vi "rad7_subviv2.vi"(8 "error in (no error)":errorcluster, 10 "Slow control read rate (Hz)":dbl=1.0, 11 "VISA resource name":refnum<visa-resource-name>) -> (0 "error out":errorcluster, 1 "Buffer length":u32, 2 "Rad7 data out":string, 3 "VISA resource name out":refnum<visa-resource-name>, 4 "Erase done?":bool)   [LabVIEW 2012]
uses:
  <vilib>/Instr/_visa.llb/VISA Configure Serial Port (Instr).vi
panel:
  out "Enum":T1(ring)
  out "Numeric 2":i32
  out "read buffer":string
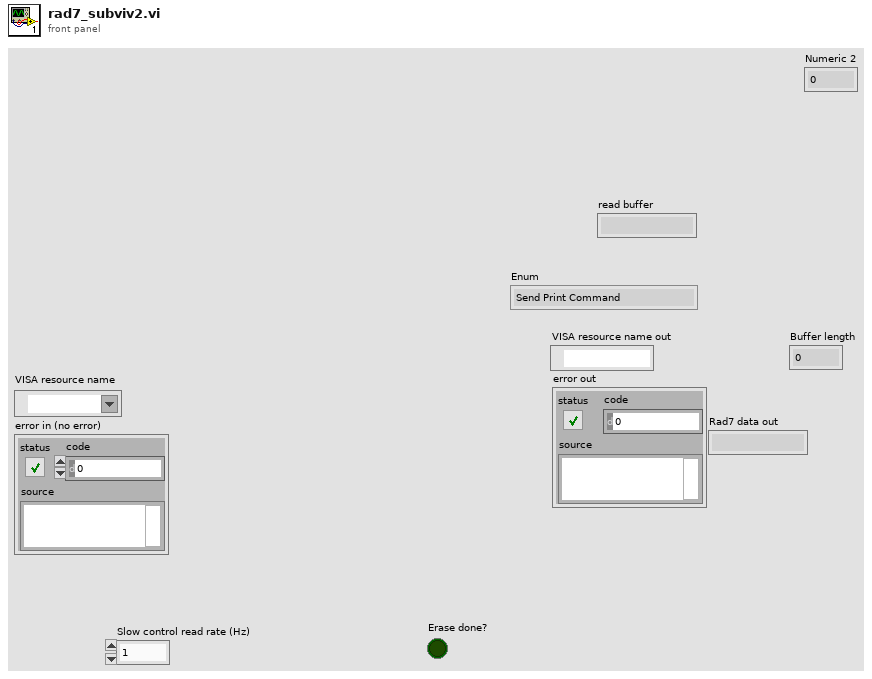
[diagram p1: front panel]
types:
  T1 = enum16{"Send Print Command", "Wait 5 seconds", "Remove first junk characters", "Data good?", "Read Buffer", "Wait 1 second", "Erase data from Rad7", "Confirm", "Error"}
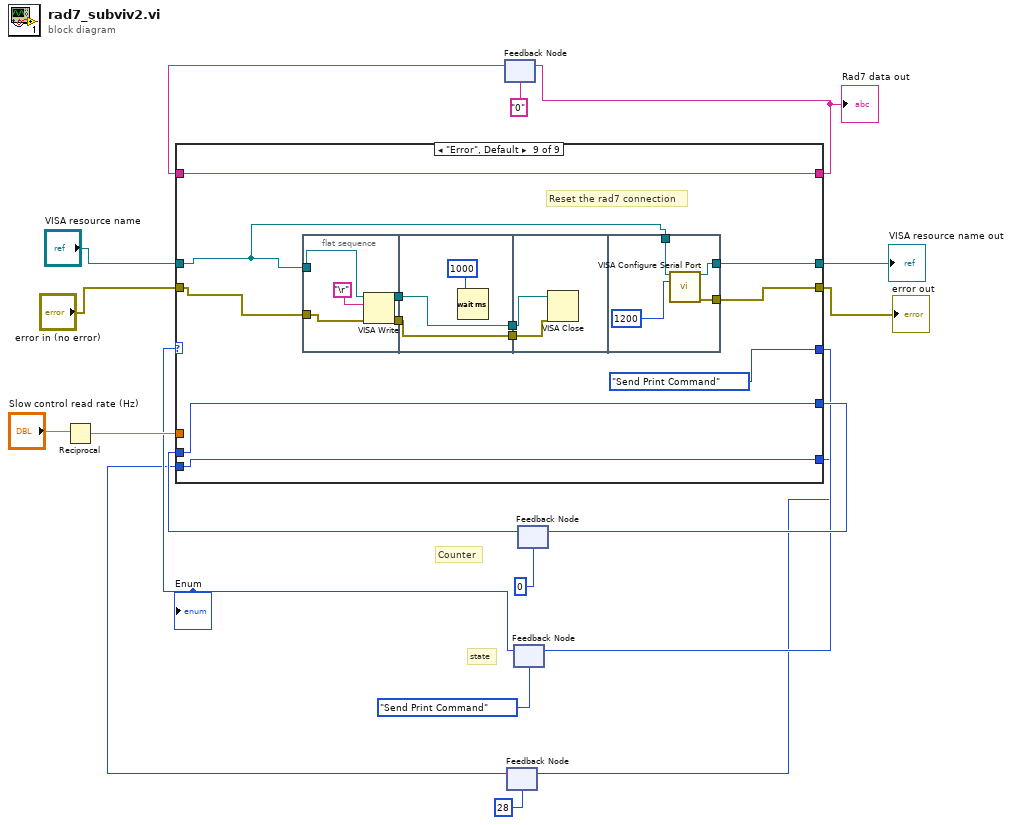
[diagram p0: block diagram]
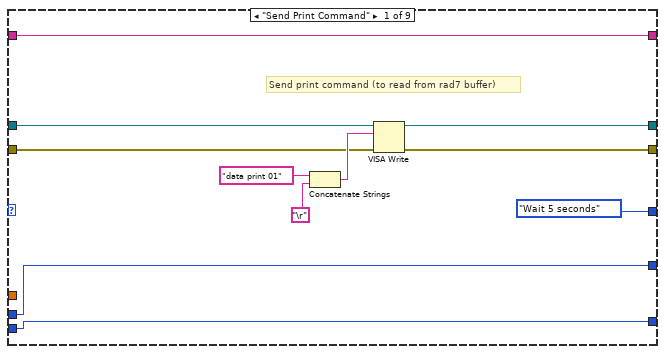
[diagram p2: hidden frame]
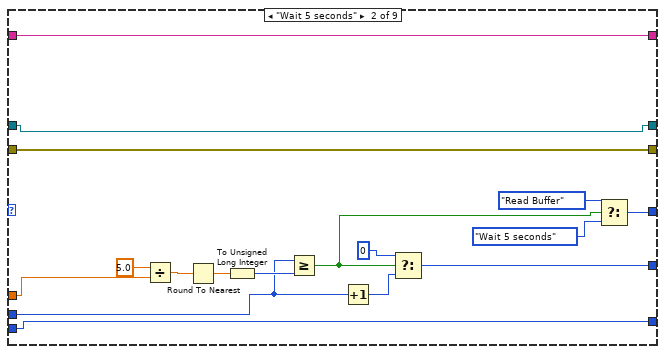
[diagram p3: hidden frame]
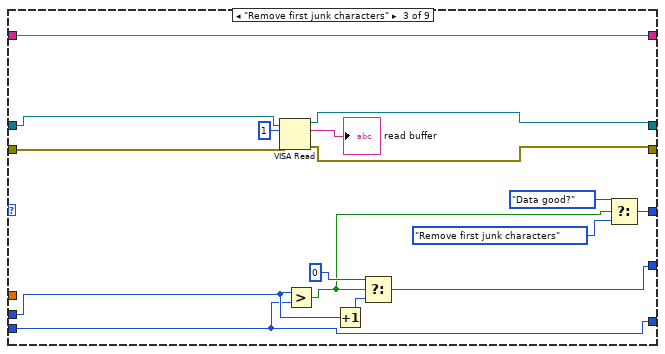
[diagram p4: hidden frame]
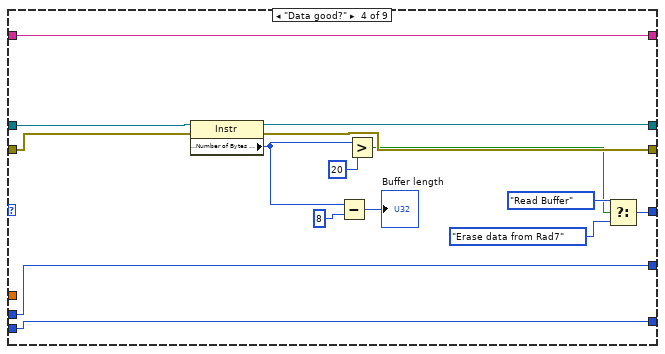
[diagram p5: hidden frame]
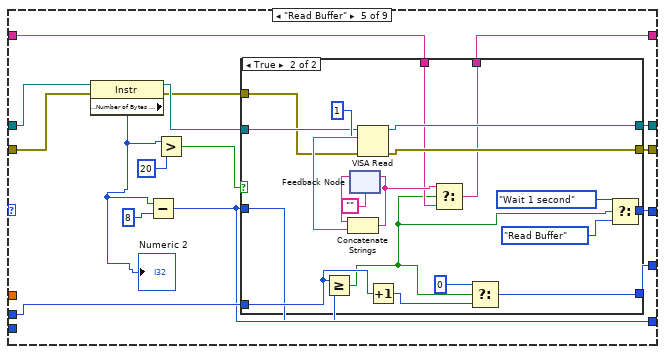
[diagram p6: hidden frame]
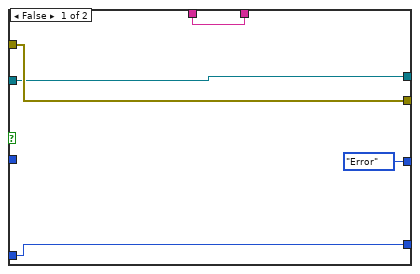
[diagram p7: hidden frame]
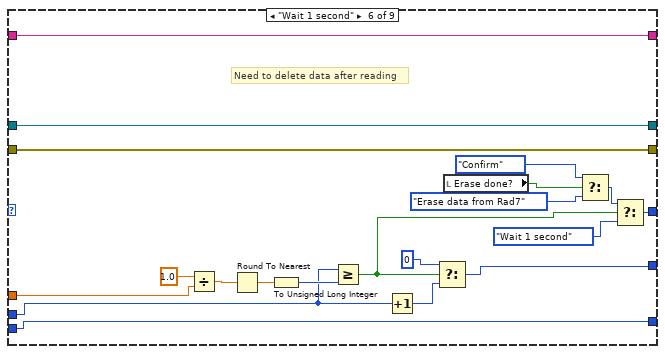
[diagram p8: hidden frame]
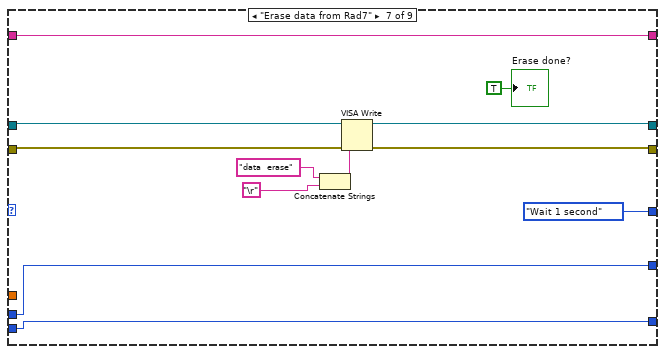
[diagram p9: hidden frame]
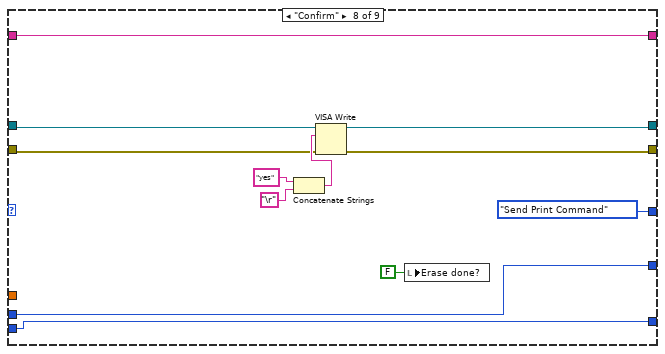
[diagram p10: hidden frame]
diagram:
  # "state"
  # "Counter"
  n1 = Reciprocal(x="Slow control read rate (Hz)") -> (1/x=w12:dbl)
  n2 = feedback #1("0") -> (w9:string)
  n3 = feedback #2(u32 28 ("y")) -> (w2:u32)
  n4 = feedback #3(T1."Send Print Command" ("Enum")) -> (w6:T1)
  "Enum" <- w6
  n5 = feedback #4(u32 0) -> (w11:u32)
  n6 = case shown="\"Error\", Default" w6 {
    tunnel: [T1."Wait 5 seconds" ("Enum") w44 w60 w75 w93 w136 T1."Wait 1 second" ("Enum") T1."Send Print Command" ("Enum") T1."Send Print Command" ("Enum")] -> w5
    tunnel: "VISA resource name" -> [w25 w32 w53 w69 w84 w125 w145 w157 w165]
    tunnel: [w24 w32 w51 w67 w92 w125 w143 w155 w164] -> w14
    tunnel: "error in (no error)" -> [w23 w31 w52 w68 w82 w124 w144 w156 w166]
    tunnel: [w22 w31 w50 w66 w91 w124 w142 w154 w163] -> w13
    tunnel: w12 -> [_ w39 _ _ _ w127 _ _ _]
    tunnel: w11 -> [w21 w37 w57 w74 w90 w130 w140 w153 w173]
    tunnel: [w21 w36 w56 w74 w89 w129 w140 w153 w173] -> w10
    tunnel: w9 -> [w20 w33 w49 w64 w87 w126 w141 w152 w172]
    tunnel: [w20 w33 w49 w64 w88 w126 w141 w152 w172] -> w8
    tunnel: w2 -> [w19 w30 w47 w63 _ w119 w139 w151 w171]
    tunnel: [w19 w30 w47 w63 w79 w119 w139 w151 w171] -> w1
    frame "Send Print Command" {
      # "Send print command (to read from rad7 buffer)"
      n7 = Concatenate Strings("data print 01" ("Command"), "\r") -> (w28:string)
      n8 = VISA Write(VISA resource name=w25, write buffer=w28, error in (no error)=w23) -> (VISA resource name out=w24:refnum<visa-resource-name>, error out=w22:errorcluster)  [unwired: 1 out]
    }
    frame "Wait 5 seconds" {
      n9 = Divide(x=5.0, y=w39) -> (x/y=w43:dbl)
      n10 = Round To Nearest(number=w43) -> (nearest integer value=w42:dbl)
      n11 = To Unsigned Long Integer(number=w42) -> (unsigned 32bit integer=w41:u32)
      n12 = Greater Or Equal?(x=w37, y=w41) -> (x >= y?=w34:bool)
      n13 = Increment(x=w37) -> (x+1=w40:u32)
      n14 = Select(t=u32 0, s=w34, f=w40) -> (s? t:f=w36:u32)
      n15 = Select(t=T1."Read Buffer" ("Enum"), s=w34, f=T1."Wait 5 seconds" ("Enum")) -> (s? t:f=w44:T1)
    }
    frame "Remove first junk characters" {
      n16 = VISA Read(VISA resource name=w53, byte count=u32 1, error in (no error)=w52) -> (VISA resource name out=w51:refnum<visa-resource-name>, read buffer=→"read buffer":string, error out=w50:errorcluster)  [unwired: 1 out]
      n17 = Greater?(x=w57, y=w47) -> (0:w48:bool)
      n18 = Increment(x=w57) -> (x+1=w59:u32)
      n19 = Select(t=u32 0, s=w48, f=w59) -> (s? t:f=w56:u32)
      n20 = Select(t=T1."Data good?" ("Enum"), s=w48, f=T1."Remove first junk characters" ("Enum")) -> (s? t:f=w60:T1)
    }
    frame "Data good?" {
      n21 = property class="Instr"(reference=w69, error in=w68) -> (reference out=w67:refnum<visa-resource-name>, error out=w66:errorcluster, "Serial Settings:Number of Bytes at Serial Port"=w71:u32)
      n22 = Subtract(x=w71, y=u32 8) -> (x-y=→"Buffer length":u32)
      n23 = Greater?(x=w71, y=u32 20) -> (0:w65:bool)
      n24 = Select(t=T1."Read Buffer" ("Enum"), s=w65, f=T1."Erase data from Rad7" ("Enum")) -> (s? t:f=w75:T1)
    }
    frame "Read Buffer" {
      n25 = property class="Instr"(reference=w84, error in=w82) -> (reference out=w83:refnum<visa-resource-name>, error out=w81:errorcluster, "Serial Settings:Number of Bytes at Serial Port"=w80:u32)
      "Numeric 2" <- w80
      n26 = Subtract(x=w80, y=8) -> (x-y=w79:u32)
      n27 = Greater?(x=w80, y=20) -> (0:w78:bool)
      n28 = case shown="True" w78 {
        tunnel: [T1."Error" ("Enum") w116] -> w93
        tunnel: [w96 w111] -> w92
        tunnel: [w97 w110] -> w91
        tunnel: w90 -> [w95 w107]
        tunnel: [w95 w106] -> w89
        tunnel: [w98 w104] -> w88
        tunnel: w87 -> [w98 w103]
        tunnel: w83 -> [w96 w101]
        tunnel: w81 -> [w97 w100]
        tunnel: w79 -> [_ w99]
        frame False {
        }
        frame True {
          n29 = Greater Or Equal?(x=w107, y=w99) -> (x >= y?=w102:bool)
          n30 = feedback #5("") -> (w114:string)
          n31 = VISA Read(VISA resource name=w101, byte count=1, error in (no error)=w100) -> (VISA resource name out=w111:refnum<visa-resource-name>, read buffer=w115:string, error out=w110:errorcluster)  [unwired: 1 out]
          n32 = Concatenate Strings(w114, w115) -> (w105:string)
          n33 = feedback-in #5(w105) -> ()
          n34 = Increment(x=w107) -> (x+1=w109:u32)
          n35 = Select(t=w105, s=w102, f=w103) -> (s? t:f=w104:string)
          n36 = Select(t=u32 0, s=w102, f=w109) -> (s? t:f=w106:u32)
          n37 = Select(t=T1."Wait 1 second" ("Enum"), s=w102, f=T1."Read Buffer" ("Enum")) -> (s? t:f=w116:T1)
        }
      }
    }
    frame "Wait 1 second" {
      # "Need to delete data after reading"
      n38 = Divide(x=1.0, y=w127) -> (x/y=w135:dbl)
      n39 = Round To Nearest(number=w135) -> (nearest integer value=w134:dbl)
      n40 = To Unsigned Long Integer(number=w134) -> (unsigned 32bit integer=w133:u32)
      n41 = Greater Or Equal?(x=w130, y=w133) -> (x >= y?=w120:bool)
      n42 = Increment(x=w130) -> (x+1=w131:u32)
      n43 = Select(t=u32 0, s=w120, f=w131) -> (s? t:f=w129:u32)
      n44 = local read "Erase done?"() -> (w121:bool)
      n45 = Select(t=T1."Confirm" ("Enum"), s=w121, f=T1."Erase data from Rad7" ("Enum")) -> (s? t:f=w137:T1)
      n46 = Select(t=w137, s=w120, f=T1."Wait 1 second" ("Enum")) -> (s? t:f=w136:T1)
    }
    frame "Erase data from Rad7" {
      n47 = Concatenate Strings("data  erase", "\r") -> (w146:string)
      n48 = VISA Write(VISA resource name=w145, write buffer=w146, error in (no error)=w144) -> (VISA resource name out=w143:refnum<visa-resource-name>, error out=w142:errorcluster)  [unwired: 1 out]
      "Erase done?" <- TRUE ("Erase done?")
    }
    frame "Confirm" {
      n49 = Concatenate Strings("yes", "\r") -> (w158:string)
      n50 = VISA Write(VISA resource name=w157, write buffer=w158, error in (no error)=w156) -> (VISA resource name out=w155:refnum<visa-resource-name>, error out=w154:errorcluster)  [unwired: 1 out]
      n51 = local write "Erase done?"(FALSE ("Erase done?")) -> ()
    }
    frame "Error", Default {
      # "Reset the rad7 connection"
      n52 = flat-sequence {
        tunnel: w166 -> [w178]
        tunnel: w165 -> [w177]
        tunnel: [w176] -> w170
        tunnel: [w175] -> w169
        tunnel: [w181] -> w168
        tunnel: w170 -> [w181]
        tunnel: [w180] -> w167
        tunnel: w169 -> [w180]
        tunnel: w168 -> [w184]
        tunnel: w167 -> [w183]
        tunnel: w165 -> [w187]
        tunnel: [w186] -> w164
        tunnel: [w185] -> w163
        frame #0 {
          n53 = VISA Write(VISA resource name=w177, write buffer="\r", error in (no error)=w178) -> (VISA resource name out=w176:refnum<visa-resource-name>, error out=w175:errorcluster)  [unwired: 1 out]
        }
        frame #1 {
          n54 = Wait (ms)(milliseconds to wait=1000) -> ()  [unwired: 1 out]
        }
        frame #2 {
          n55 = VISA Close(VISA resource name=w184, error in (no error)=w183) -> ()  [unwired: 1 out]
        }
        frame #3 {
          n56 = call-poly "VISA Configure Serial Port"("VISA resource name"=w187, "baud rate (9600)"=1200) -> ("VISA resource name out"=w186:refnum<visa-resource-name>, "error out"=w185:errorcluster)  [unwired: 12 in]
        }
      }
    }
  }
  "error out" <- w13
  "VISA resource name out" <- w14
  "Rad7 data out" <- w8
  n57 = feedback-in #1(w8) -> ()
  n58 = feedback-in #2(w1) -> ()
  n59 = feedback-in #3(w5) -> ()
  n60 = feedback-in #4(w10) -> ()
